vi "IsOuterTerminal.vi"(5 "terminal":refnum<class "Terminal.lvclass">, 6 "error in":errorcluster, 9 "Tunnel in":refnum<class "Tunnel.lvclass">) -> (0 "error out":errorcluster, 3 "Tunnel out":refnum<class "Tunnel.lvclass">, 4 "Outer":bool)   [LabVIEW 2014, in "Tunnel.lvclass"]
uses:
  Tunnel.lvclass
  Terminal/Terminal.lvclass
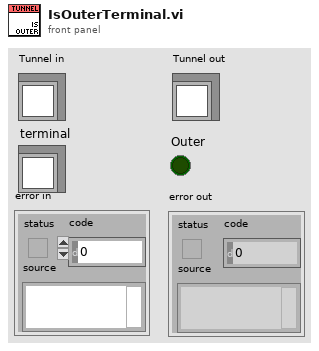
[diagram p1: front panel]
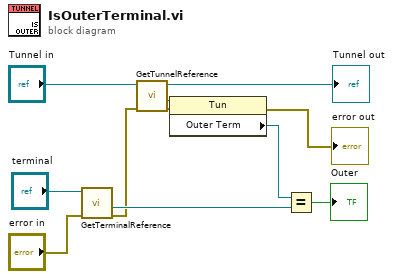
[diagram p0: block diagram]
diagram:
  n1 = call "GetTerminalReference.vi"("error in"="error in", "Terminal in"="terminal") -> ("error out"=w2:errorcluster, "reference"=w4:refnum<vi>)  [unwired: 7 in, 1 out]
  n2 = call "GetTunnelReference.vi"("error in"=w2, "Tunnel in"="Tunnel in") -> ("error out"=w10:errorcluster, "reference out"=w9:refnum<vi>, "Tunnel out"=→"Tunnel out":refnum<class "Tunnel.lvclass">)  [unwired: 7 in]
  n3 = property class="Tun"(reference=w9, error in=w10) -> (error out=→"error out":errorcluster, "Outer Term"=w5:refnum<vi>)  [unwired: 1 out]
  n4 = Equal?(x=w5, y=w4) -> (x = y?=→"Outer":bool)
